vi "KEN.vi"(0 "System no.":i32=1 min=1 max=4 step=1, 1 "Name":string, 5 "error in":errorcluster) -> (14 "Controller error":bool, 19 "error out":errorcluster)   [LabVIEW 2020]
doc: "Activates an already defined coordinate system; i.e. assigns \"active\" state and queries ERR?. KEN sets the pivot point coordinates (\"SPI.vi\") to zero when a KSD, KSW or KST coordinate system is active. Activating KLF, KLD, KSB or KSF does not change the pivot point settings. If the hexapod is moving, the command cannot be applied. Activating coordinate systems of type KLD, KLF and KSB requires command level 1 (CCL.vi). KEN settings are volatile but can be saved as power-on default with WPA.vi using the password \"SKS\". Controller error is TRUE if selected system reports error code not equal to 0.\n\nC-887, F-206, M-8X0: Only for GCS syntax version = GCS 2.0 or higher (Check with CSV?.vi. If CSV?.vi is not supported, syntax version is GCS 1.0)."
panel:
  # "Enables an already defined coordinate system; i.e. \nassigns \"enabled\" state. and queries ERR?."
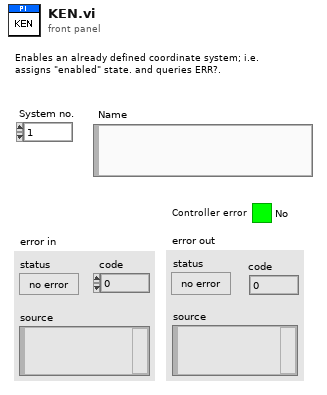
[diagram p1: front panel]
types:
  T1 = enum16{"Disable error check", "Force error check", "Use global settings"}
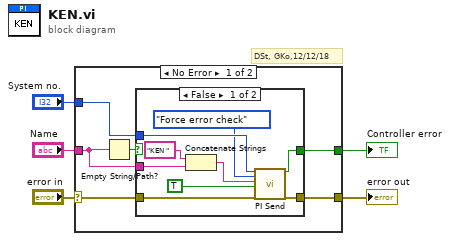
[diagram p0: block diagram]
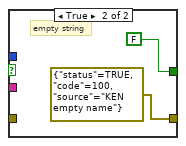
[diagram p2: hidden frame]
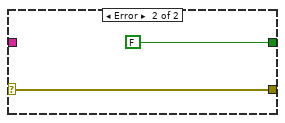
[diagram p3: hidden frame]
diagram:
  # "DSt, GKo,12/12/18"
  n1 = case shown="No Error" "error in" {
    selector: "error in" -> [w8 w23]
    tunnel: [w11 w23] -> w5
    tunnel: [w10 FALSE ("Controller error")] -> w4
    tunnel: "System no." -> [w9 _]
    tunnel: "Name" -> [w7 _]
    frame No Error {
      n2 = Empty String/Path?(string/path=w7) -> (empty?=w6:bool)
      n3 = case shown="False" w6 {
        tunnel: w8 -> [w20 _]
        tunnel: [w15 errorcluster {"status"=TRUE, "code"=100, "source"="KEN empty name"} ("error out")] -> w11
        tunnel: [w14 FALSE ("Controller error")] -> w10
        tunnel: w9 -> [w17 _]
        tunnel: w7 -> [w16 _]
        frame False {
          n4 = Concatenate Strings("KEN ", w16) -> (w18:string)
          n5 = call "PI Send.vi"("System no."=w17, "Error check settings"=T1."Force error check", "String to send"=w18, "Attach termination char.?"=TRUE ("Attach Linefeed?"), "error in"=w20) -> ("Controller error"=w14:bool, "error out"=w15:errorcluster)  [unwired: 1 in, 12 out]
        }
        frame True {
          # "empty string"
        }
      }
    }
    frame Error {
    }
  }
  "error out" <- w5
  "Controller error" <- w4
